vi "Get Count Convert Wavelength Range.vi"(8 "error in (no error)":errorcluster, 10 "maxval":sgl, 11 "minval":sgl) -> (0 "error out":errorcluster, 1 "function return":u32, 2 "maxval out":sgl, 3 "minval out":sgl)   [LabVIEW 2014, in "atmcd32d.lvlib"]
doc: "unsigned int WINAPI GetCountConvertWavelengthRange(float * minval, float * maxval);"
uses:
  atmcd32d.lvlib
  atmcd32d.dll
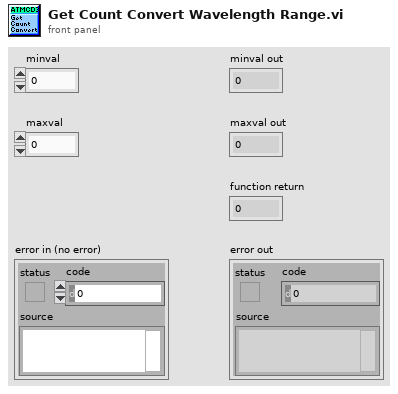
[diagram p1: front panel]
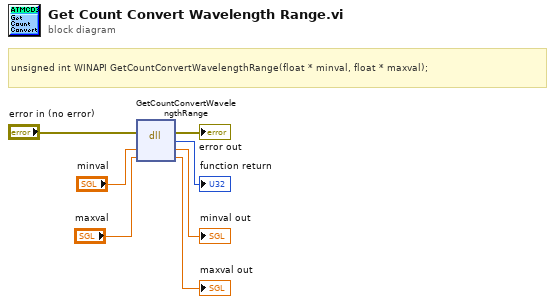
[diagram p0: block diagram]
diagram:
  # "unsigned int WINAPI GetCountConvertWavelengthRange(float * minval, float * maxval);"
  n1 = dll-call lib="C:/Users/Bakir/Documents/Lambda2-Testing/lib/Andorlib/atmcd32d.*" fn="GetCountConvertWavelengthRange"(error in="error in (no error)", "minval"="minval", "maxval"="maxval") -> (error out=→"error out":errorcluster, →"function return":u32, "minval"=→"minval out":sgl, "maxval"=→"maxval out":sgl)  [unwired: 2 in, 1 out]
